vi "Vision Processing.vi"(4 "error in (no error)":errorcluster) -> ()   [LabVIEW 2019]
doc: "This VI runs in parallel to other tasks. It gets images from the camera, processes them for color or shape and uses commands or globals to affect the behavior of other subsystems."
uses:
  Framework/Robot Global Data.vi
  <vilib>/vision/NI_Vision_Development_Module.lvlib
panel:
  out "Results":T1(array[cluster]) {"Normalized Center"."x" format="%#_2g"; "Normalized Center"."y" format="%#_2g"; "Overall Score" format="%#_2g"; "Distance (ft)" format="%#_3g"; "Area Score" format="%#_2g"; "Moment Score" format="%#_2g"; "Aspect Score" format="%#_2g"}
  in  "Size Limit %":dbl=0.1 min=0.0 max=100.0 step=0.01 format="%#_13g"
  in  "Particle Count LImit":i32=5
  out "Qualified":i32
  out "Mask":T2(plugin-control)
  out "Original Image":T2(plugin-control)
  # "Scores"
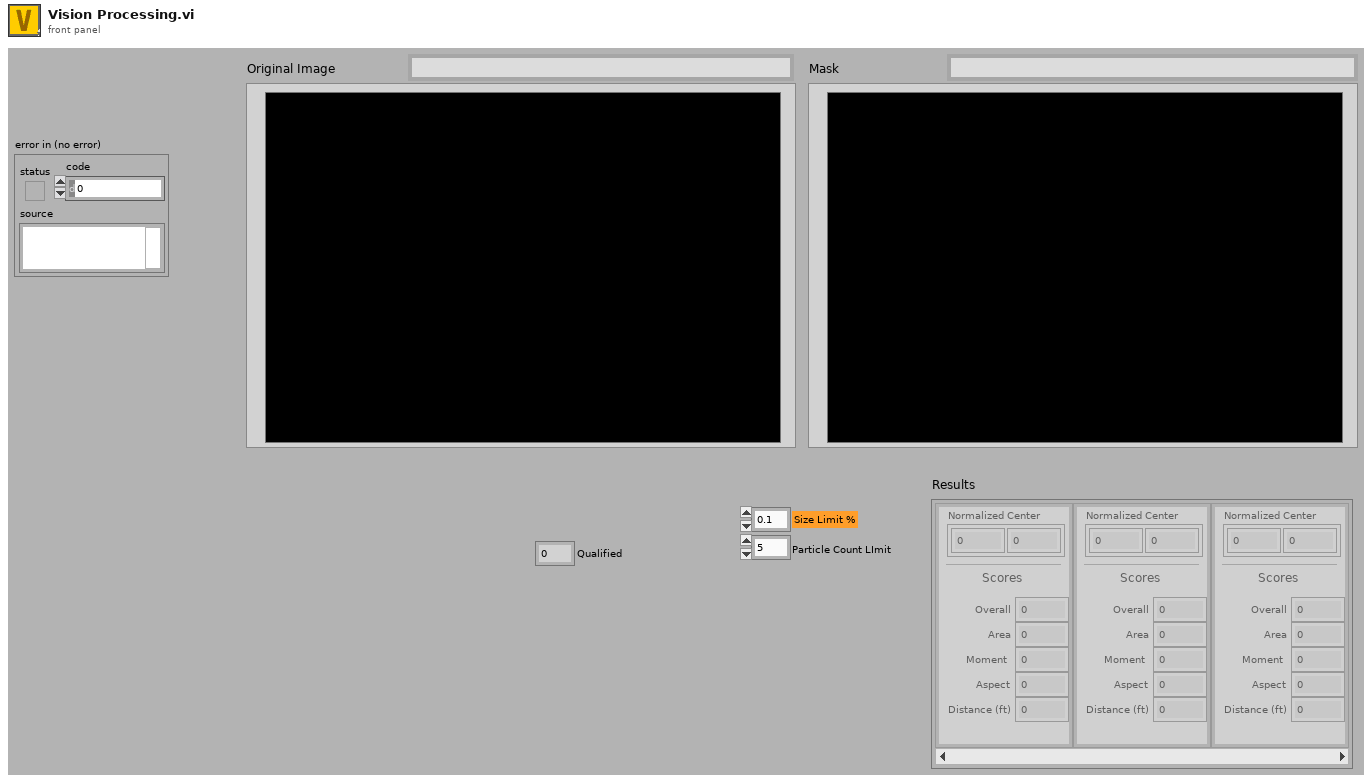
[diagram p1: front panel]
types:
  T1 = cluster{"diameter points":cluster{"first point":cluster{"x":dbl, "y":dbl}, "projected point":cluster{"x":dbl, "y":dbl}}, "Normalized Center":cluster{"x":dbl, "y":dbl}, "Overall Score":dbl, "Area Score":dbl, "Moment Score":dbl, "Aspect Score":dbl, "Distance (ft)":dbl, "Upper Goal":bool}[]
  T2 = typedef "IMAQ Image.ctl" = refnum<image>
  T3 = typedef "Particle Parameters" = i32
  T4 = cluster{"Hue":cluster{dbl, dbl}, "Sat":cluster{dbl, dbl}, "Val":cluster{dbl, dbl}}
  T5 = typedef "Target Fields.ctl" = cluster{"diameter points":cluster{"first point":cluster{"x":dbl, "y":dbl}, "projected point":cluster{"x":dbl, "y":dbl}}, "normalized center":cluster{"x":dbl, "y":dbl}, "Overall Score":dbl, "Area Score":dbl, "Moment Score":dbl, "Aspect Score":dbl, "Distance (ft)":dbl, "Upper Goal":bool}
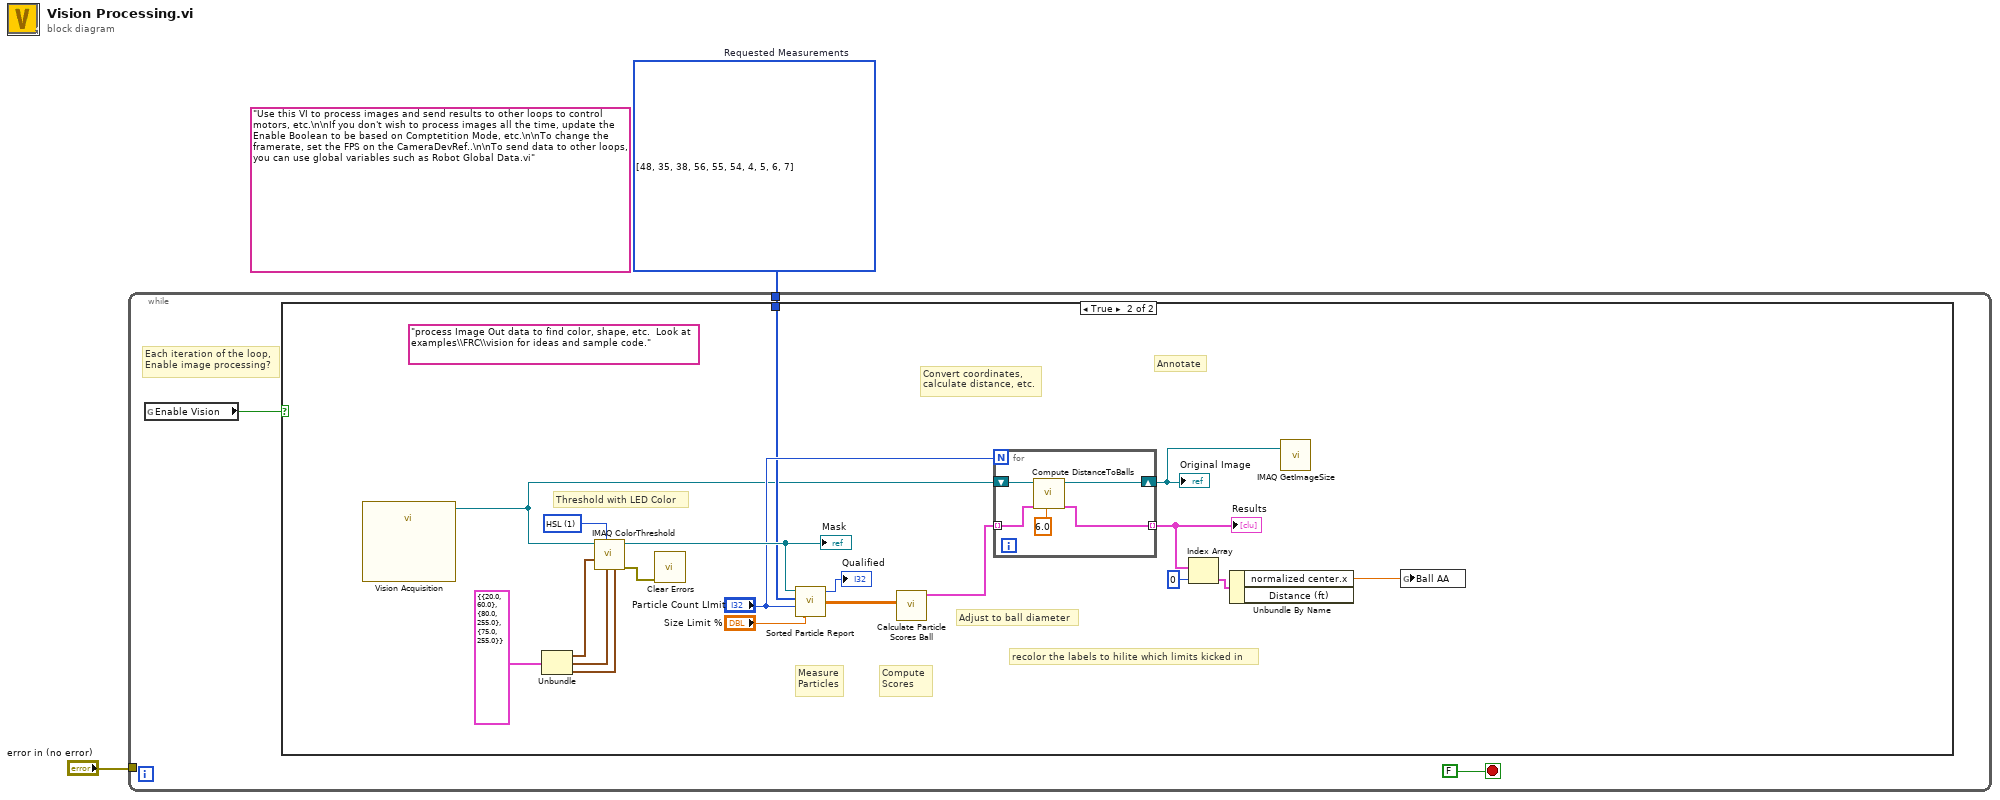
[diagram p0: block diagram]
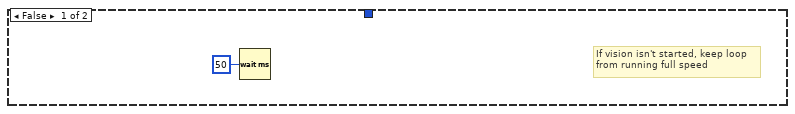
[diagram p2: hidden frame]
diagram:
  w1 = T3[] [48, 35, 38, 56, 55, 54, 4, 5, 6, 7] items=["Center of Mass X", "Center of Mass Y", "First Pixel X", "First Pixel Y", "Bounding Rect Left", "Bounding Rect Top", "Bounding Rect Right", "Bounding Rect Bottom", "Max Feret Diameter Start X", "Max Feret Diameter Start Y", "Max Feret Diameter End X", "Max Feret Diameter End Y", "Max Horiz. Segment Length Left", "Max Horiz. Segment Length Right", "Max Horiz. Segment Length Row", "-", "Bounding Rect Width", "Bounding Rect Height", "Bounding Rect Diagonal", "Perimeter", "Convex Hull Perimeter", "Holes' Perimeter", "Max Feret Diameter", "Equivalent Ellipse Major Axis", "Equivalent Ellipse Minor Axis", "Equivalent Ellipse Minor Axis (Feret)", "Equivalent Rect Long Side", "Equivalent Rect Short Side", "Equivalent Rect Diagonal", "Equivalent Rect Short Side (Feret)", "Average Horiz. Segment Length", "Average Vert. Segment Length", "Hydraulic Radius", "Waddel Disk Diameter", "-", "Area", "Holes' Area", "Particle & Holes' Area", "Convex Hull Area", "Image Area", "-", "Number of Holes", "Number of Horiz. Segments", "Number of Vert. Segments", "-", "Orientation", "Max Feret Diameter Orientation", "-", "% Area/Image Area", "% Area/(Particle & Holes' Area)", "Ratio of Equivalent Ellipse Axes", "Ratio of Equivalent Rect Sides", "-", "Elongation Factor", "Compactness Factor", "Heywood Circularity Factor", "Type Factor", "-", "Sum X", "Sum Y", "Sum XX", "Sum XY", "Sum YY", "Sum XXX", "Sum XXY", "Sum XYY", "Sum YYY", "-", "Moment of Inertia XX", "Moment of Inertia XY", "Moment of Inertia YY", "Moment of Inertia XXX", "Moment of Inertia XXY", "Moment of Inertia XYY", "Moment of Inertia YYY", "Norm. Moment of Inertia XX", "Norm. Moment of Inertia XY", "Norm. Moment of Inertia YY", "Norm. Moment of Inertia XXX", "Norm. Moment of Inertia XXY", "Norm. Moment of Inertia XYY", "Norm. Moment of Inertia YYY", "Hu Moment 1", "Hu Moment 2", "Hu Moment 3", "Hu Moment 4", "Hu Moment 5", "Hu Moment 6", "Hu Moment 7"]  # Requested Measurements
  (unwired) "Use this VI to process images and send results to other loops to control motors, etc.\n\nIf you don't wish to process images all the time, update the Enable Boolean to be based on Comptetition Mode, etc.\n\nTo change the framerate, set the FPS on the CameraDevRef..\n\nTo send data to other loops, you can use global variables such as Robot Global Data.vi"
  n1 = while {
    tunnel: "error in (no error)" -> [_]
    tunnel: w1 -> [w3]
    stop <- FALSE stop-if-true
    # "Each iteration of the loop,\nEnable image processing?"
    n2 = global read "Robot Global Data.vi" "Enable Vision"() -> (w4:bool)
    n3 = case shown="True" w4 {
      tunnel: w3 -> [_ w15]
      frame False {
        # "If vision isn't started, keep loop\nfrom running full speed"
        n4 = Wait (ms)(milliseconds to wait=u32 50) -> ()  [unwired: 1 out]
      }
      frame True {
        w14 = u16 1 items=["RGB", "HSL", "HSV", "HSI"] ("Color Mode")
        (unwired) "process Image Out data to find color, shape, etc.  Look at examples\\FRC\\vision for ideas and sample code."
        # "recolor the labels to hilite which limits kicked in"
        # "Adjust to ball diameter"
        # "Measure\nParticles"
        # "Convert coordinates,\ncalculate distance, etc."
        # "Annotate"
        # "Compute\nScores"
        # "Threshold with LED Color"
        n5 = call "Vision Acquisition"() -> ("Image Out"=w9:T2)  [unwired: 25 in, 2 out]
        n6 = Unbundle(T4 {"Hue"={20.0, 60.0}, "Sat"={80.0, 255.0}, "Val"={75.0, 255.0}} ("cluster")) -> ("Hue"=w25:cluster{dbl, dbl}, "Sat"=w24:cluster{dbl, dbl}, "Val"=w23:cluster{dbl, dbl})
        n7 = call "IMAQ ColorThreshold"("Blue or Luma or Val or Inten Range"=w23, "Green or Sat Range"=w24, "Color Mode"=w14, "Red or Hue Range"=w25, "Image Src"=w9) -> ("error out"=w19:errorcluster, "Image Dst Out"=w20:T2)  [unwired: 5 in]
        "Mask" <- w20
        n8 = call <vilib>:"Clear Errors.vi"("error in (no error)"=w19) -> ()  [unwired: 5 in, 2 out]
        n9 = call "Sorted Particle Report.vi"("Min Area Size %"="Size Limit %", "Particle Count Limit"="Particle Count LImit", "Pixel Measurements"=w15, "Image in"=w20) -> ("Sorted Data"=w18:dbl[][], "Particles"=→"Qualified":i32)  [unwired: 1 out]
        n10 = call "Calculate Particle Scores Ball.vi"("Sorted Data"=w18) -> ("Scores"=w17:T5[])  [unwired: 10 in]
        n11 = for {
          N: "Particle Count LImit" -> [_]
          tunnel: w17 -> [w30] mode=indexing
          shift-right: [w26] -> w8
          shift-left: w9 -> [w28]
          tunnel: [w29] -> w12 mode=indexing
          n12 = call "Compute DistanceToBalls.vi"("Target Width (in)"=6.0, "results"=w30, "Image Src"=w28) -> ("results out"=w29:T5, "Image Dst Out"=w26:T2)  [unwired: 7 in]
        }
        "Original Image" <- w8
        "Results" <- w12
        n13 = Index Array(array=w12, index=0) -> (element=w10:T5)
        n14 = Unbundle By Name(w10) -> ("normalized center.x"=w7:dbl)  [unwired: 1 out]
        n15 = call "IMAQ GetImageSize"("Image"=w8) -> ()  [unwired: 3 in, 3 out]
        n16 = global write "Robot Global Data.vi" "Ball AA"(w7) -> ()
      }
    }
  }
